vi "8Q_backtrace2.vi"(10 "all_x":i32[](array[numeric]), 11 "BT_bfr":i32[](array[numeric])=[4, 2]) -> (0 "<0_stop":bool, 2 "next_start":i32[](array[numeric]), 3 "BT_result":i32[](array[numeric]))   [LabVIEW 2012]
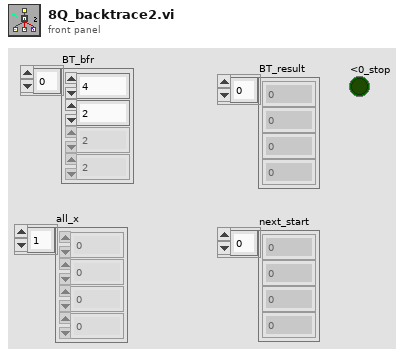
[diagram p1: front panel]
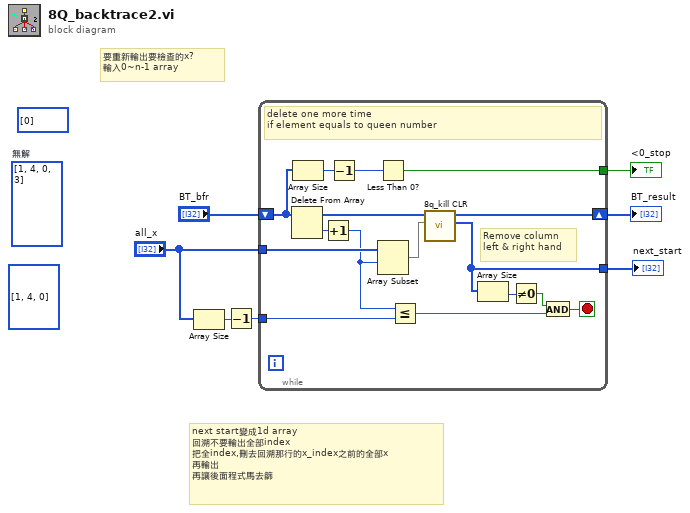
[diagram p0: block diagram]
diagram:
  (unwired) i32[] [1, 4, 0]
  (unwired) i32[] [0]
  (unwired) i32[] [1, 4, 0, 3]  # 無解
  # "next start變成1d array\n回溯不要輸出全部index\n把全index,刪去回溯那行的x_index之前的全部x\n再輸出\n再讓後面程式馬去篩"
  # "要重新輸出要檢查的x?\n輸入0~n-1 array"
  n1 = Array Size(array="all_x") -> (size(s)=w3:i32)
  n2 = Decrement(x=w3) -> (x-1=w4:i32)
  n3 = while {
    tunnel: [w21] -> w7
    tunnel: w4 -> [w20]
    shift-right: [w14] -> w6
    shift-left: "BT_bfr" -> [w19]
    tunnel: "all_x" -> [w18]
    tunnel: [w12] -> w1
    stop <- w8 stop-if-true
    # "Remove column\nleft & right hand"
    # "delete one more time\nif element equals to queen number"
    n4 = Delete From Array(array=w19) -> (deleted portion=w17:i32, array with subset deleted=w15:i32[])  [unwired: 2 in]
    n5 = Array Size(array=w19) -> (size(s)=w23:i32)
    n6 = Increment(x=w17) -> (x+1=w16:i32)
    n7 = Decrement(x=w23) -> (x-1=w22:i32)
    n8 = Less Than 0?(x=w22) -> (x < 0?=w21:bool)
    n9 = Array Subset(array=w18, index=w16) -> (w13:i32[])  [unwired: 1 in]
    n10 = Less Or Equal?(x=w16, y=w20) -> (x <= y?=w9:bool)
    n11 = call "8q_kill CLR.vi"("nextX in"=w13, "queen in"=w15) -> ("nextX"=w12:i32[], "queen"=w14:i32[])  [unwired: 8 in]
    n12 = Array Size(array=w12) -> (size(s)=w11:i32)
    n13 = Not Equal To 0?(x=w11) -> (x != 0?=w10:bool)
    n14 = And(x=w10, y=w9) -> (x .and. y?=w8:bool)
  }
  "BT_result" <- w6
  "<0_stop" <- w7
  "next_start" <- w1
